vi "Load Sub Panel.vi"(8 "error in (no error)":errorcluster, 11 "[V] Waveform in":refnum<class "[V] Waveform.lvclass">) -> (0 "error out":errorcluster, 3 "[V] Waveform out":refnum<class "[V] Waveform.lvclass">)   [LabVIEW 2023, in "[V] Waveform.lvlib" / "[V] Waveform.lvclass"]
uses:
  [V] Waveform.lvclass
  [V] Waveform.lvclass/[V] Waveform.ctl
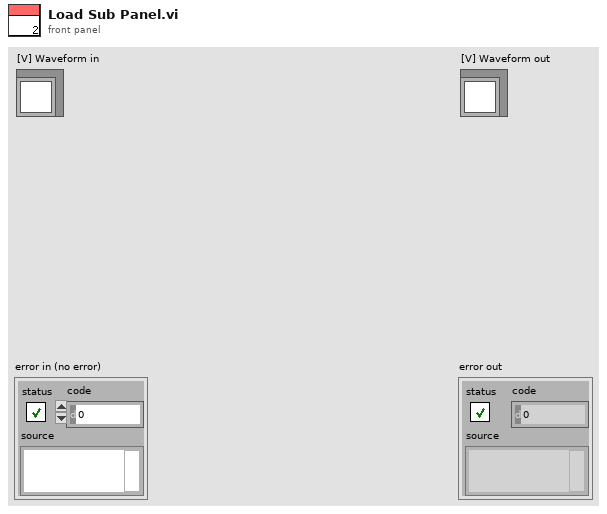
[diagram p1: front panel]
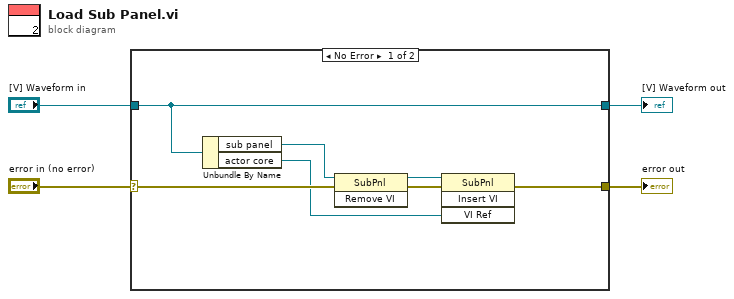
[diagram p0: block diagram]
diagram:
  n1 = case shown="No Error" "error in (no error)" {
    selector: "error in (no error)" -> [w10 w13]
    tunnel: [w6 w13] -> w3
    tunnel: [w11 w12] -> w1
    tunnel: "[V] Waveform in" -> [w11 w12]
    frame No Error {
      n2 = Unbundle By Name(w11) -> ("sub panel"=w5:refnum<vi>, "actor core"=w7:refnum<vi>)
      n3 = invoke class="SubPnl" method="Remove VI"(reference=w5, error in=w10) -> (reference out=w8:refnum<vi>, error out=w9:errorcluster)  [unwired: 1 in, 1 out]
      n4 = invoke class="SubPnl" method="Insert VI"(reference=w8, error in=w9, "VI Ref"=w7) -> (error out=w6:errorcluster)  [unwired: 1 in, 3 out]
    }
    frame Error {
    }
  }
  "error out" <- w3
  "[V] Waveform out" <- w1
